vi "VisionTracking.vi"(0 "Refnum in":T1, 5 "Range":cluster{"Lower value":sgl, "Upper value":sgl}={"Lower value"=150.0, "Upper value"=255.0} {"Lower value" scale=0.0..255.0; "Upper value" scale=0.0..255.0}, 7 "Score Limits":T2={"Rect Coverage"=60.0, "X Edge Strength"=40.0, "Y Edge Strength"=60.0, "Center"=75.0, "Outer"=75.0}, 12 "New Image 2":T1, 13 "New Image":T1) -> (4 "Refnum out":T1(plugin-control), 8 "Out Target Info":cluster{"X":dbl, "Y":dbl, "Distance (ft)":dbl}, 10 "Out Cirlcle Info":cluster{"X":dbl, "Y":dbl})   [LabVIEW 2012]
uses:
  <vilib>/vision/Image Controls.llb/IMAQ Image.ctl
  <vilib>/vision/NI_Vision_Development_Module.lvlib
panel:
  out "Circle Info":cluster{dbl, dbl, dbl}[](array[cluster])
  in  "Color Plane":i32(ring)=6 items=["Red", "Green", "Blue", "Hue", "Saturation", "Luminance", "Value", "Intensity"]
  in  "Area Size Limit %":dbl=0.5
  in  "Particle Count Limit":i32=10
  in  "Camera Type":enum16{"206", "1011", "1013"}(ring)
  out "Target Info":T3(array[cluster])
  in  "Annotate":bool=TRUE
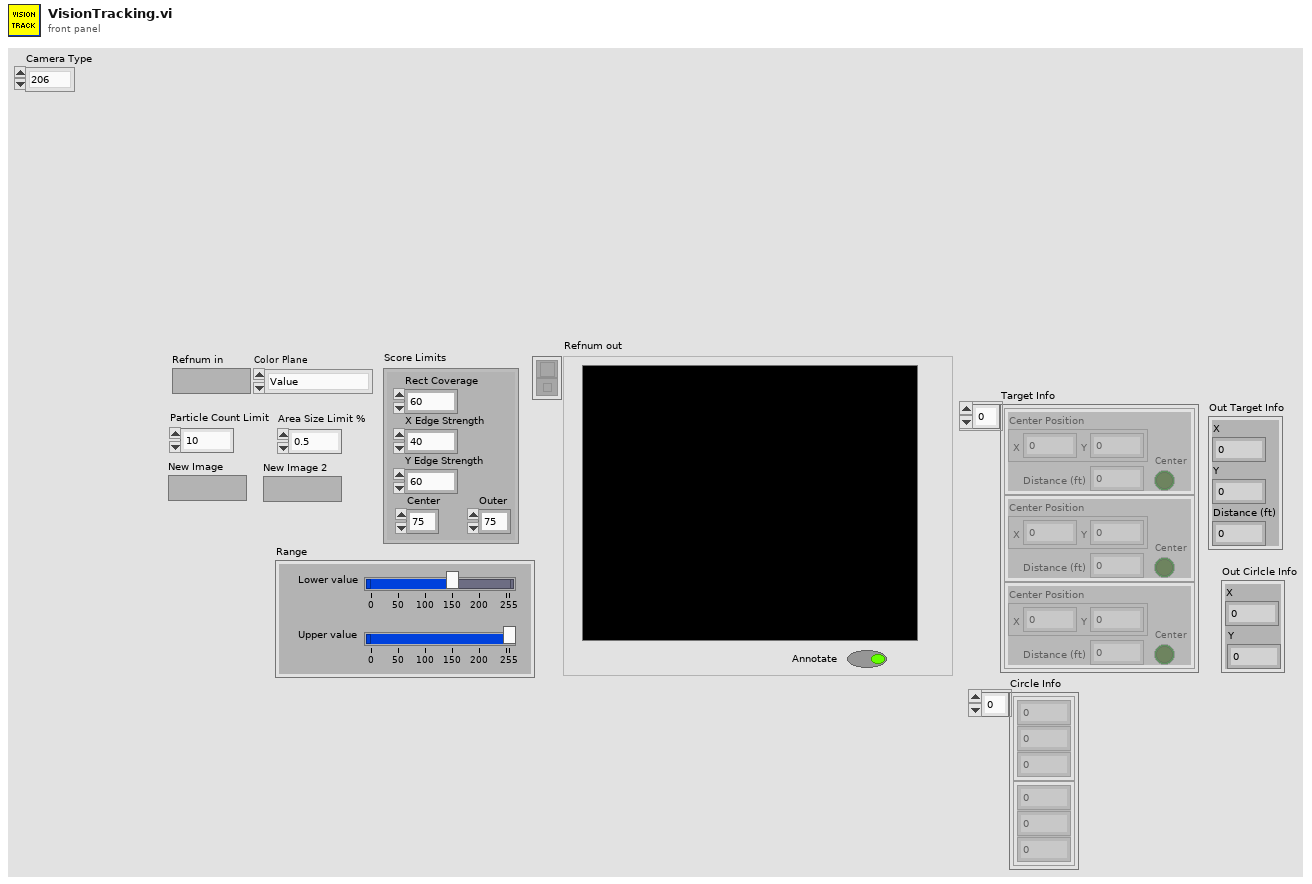
[diagram p1: front panel]
types:
  T1 = typedef "IMAQ Image.ctl" = refnum<image>
  T2 = cluster{"Rect Coverage":dbl, "X Edge Strength":dbl, "Y Edge Strength":dbl, "Center":dbl, "Outer":dbl}
  T3 = cluster{"Center Position":cluster{"X":dbl, "Y":dbl}, "Distance (ft)":dbl, "Center":bool}[]
  T4 = cluster{"Position":cluster{"X":dbl, "Y":dbl}, "Distance (ft)":dbl, bool}[]
  T5 = cluster{cluster{"Left":dbl, "Top":dbl, "Right":dbl, "Bottom":dbl}, "Scores":dbl[], cluster{"Long":dbl, "Short":dbl}}[]
  T6 = cluster{"Target Center (-1 to 1)":cluster{"X":dbl, "Y":dbl}, "Distance (ft)":dbl, "Center Target":bool}
  T7 = cluster{"Target Center (-1 to 1)":cluster{"X":dbl, "Y":dbl}, "Distance (ft)":dbl, "Center Target":bool}[]
  T8 = cluster{"Left":dbl, "Top":dbl, "Right":dbl, "Bottom":dbl}
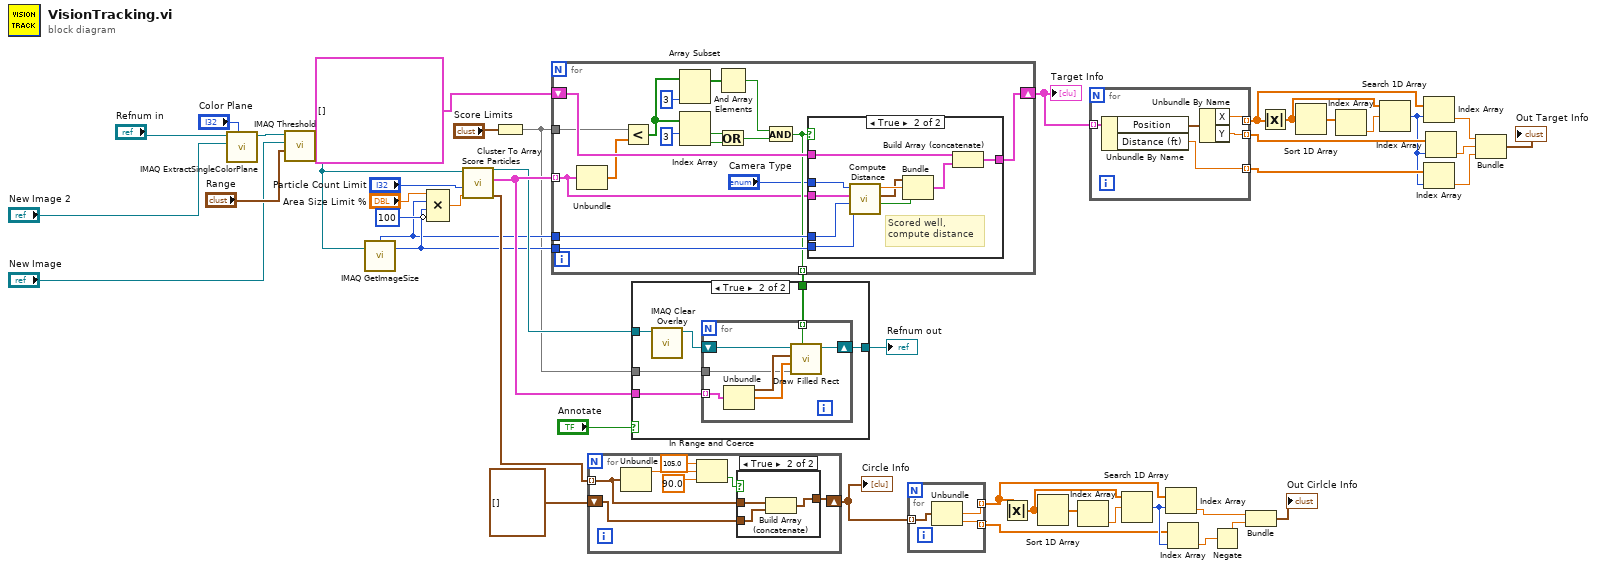
[diagram p0: block diagram]
diagram:
  n1 = call "IMAQ ExtractSingleColorPlane"("Color Plane"="Color Plane", "Image Dst"="New Image 2", "Image Src"="Refnum in") -> ("Image Dst Out"=w14:T1)  [unwired: 1 in, 7 out]
  n2 = call "IMAQ Threshold"("Range"="Range", "Image Dst"="New Image", "Image Src"=w14) -> ("Image Dst Out"=w19:T1)  [unwired: 3 in, 5 out]
  n3 = call "IMAQ GetImageSize"("Image"=w19) -> ("Y Resolution"=w12:i32, "X Resolution"=w11:i32)  [unwired: 3 in, 1 out]
  n4 = Compound Arithmetic op=MULTIPLY("Area Size Limit %", w11, w12, invert 100 ("value")) -> (w17:dbl)
  n5 = call "Score Particles.vi"("Area Size Limit"=w17, "Particle Count Limit"="Particle Count Limit", "Image Refnum in"=w19) -> ("Circle Info"=w23:cluster{dbl, dbl, dbl}[], "Scored Particle Info"=w21:T5, "Image Refnum out"=w20:T1)  [unwired: 6 in]
  n6 = Cluster To Array(cluster="Score Limits") -> (array=w7:dbl[])
  n7 = for {
    shift-right: [w62] -> w45
    shift-left: T4 [] -> [w63]
    tunnel: w11 -> [w61]
    tunnel: w21 -> [w48] mode=indexing
    tunnel: w7 -> [w59]
    tunnel: w12 -> [w58]
    tunnel: [w49] -> w8 mode=indexing
    n8 = Unbundle(w48) -> ("Scores"=w60:dbl[])  [unwired: 2 out]
    n9 = Less?(x=w59, y=w60) -> (x < y?=w55:bool[])
    n10 = Array Subset(array=w55, length=3) -> (w56:bool[])  [unwired: 1 in]
    n11 = Index Array(array=w55, index #1=3 ("length")) -> (element #1=w53:bool, element #2=w52:bool)  [unwired: 1 in]
    n12 = And Array Elements(Boolean array=w56) -> (logical AND=w50:bool)
    n13 = Or(x=w53, y=w52) -> (x .or. y?=w51:bool)
    n14 = And(x=w50, y=w51) -> (x .and. y?=w49:bool)
    n15 = case shown="True" w49 {
      tunnel: w63 -> [w64 w74]
      tunnel: [w64 w73] -> w62
      tunnel: w61 -> [_ w71]
      tunnel: w58 -> [_ w68]
      tunnel: w48 -> [_ w67]
      tunnel: "Camera Type" -> [_ w65]
      frame False {
        # "Didn't score well enough"
      }
      frame True {
        # "Scored well,\ncompute distance"
        n16 = call "Compute Distance.vi"("Y Image Resolution"=w68, "X Image Resolution"=w71, "Particle Scores"=w67, "Camera Type"=w65) -> ("Center Target"=w66:bool, "Target Center (-1 to 1)"=w69:cluster{"X":dbl, "Y":dbl}, "Distance (ft)"=w70:dbl)  [unwired: 5 in]
        n17 = Bundle("Target Center (-1 to 1)"=w69, "Distance (ft)"=w70, "Center Target"=w66) -> (w72:T6)  [unwired: 1 in]
        n18 = Build Array (concatenate)(w74, w72) -> (w73:T7)
      }
    }
  }
  "Target Info" <- w45
  n19 = for {
    tunnel: w23 -> [w77] mode=indexing
    shift-right: [w75] -> w46
    shift-left: cluster{dbl, dbl, dbl}[] [] ("Circle Info") -> [w76]
    n20 = Unbundle(w77) -> (w81:dbl)  [unwired: 2 out]
    n21 = In Range and Coerce(upper limit=105.0, x=w81, lower limit=90.0) -> (In Range?=w78:bool)  [unwired: 1 out]
    n22 = case shown="True" w78 {
      tunnel: w77 -> [_ w85]
      tunnel: w76 -> [w82 w84]
      tunnel: [w82 w83] -> w75
      frame False {
      }
      frame True {
        n23 = Build Array (concatenate)(w85, w84) -> (w83:cluster{dbl, dbl, dbl}[])
      }
    }
  }
  "Circle Info" <- w46
  n24 = case shown="True" "Annotate" {
    tunnel: w20 -> [w86 w92]
    tunnel: [w86 w91] -> w4
    tunnel: w21 -> [_ w89]
    tunnel: w7 -> [_ w88]
    tunnel: w8 -> [_ w87]
    frame False {
    }
    frame True {
      n25 = call "IMAQ Clear Overlay"("Image"=w92) -> ("Image Out"=w90:T1)  [unwired: 2 in, 8 out]
      n26 = for {
        shift-right: [w98] -> w91
        shift-left: w90 -> [w99]
        tunnel: w89 -> [w95] mode=indexing
        tunnel: w88 -> [w94]
        tunnel: w87 -> [w93] mode=indexing
        n27 = Unbundle(w95) -> (w96:T8, "Scores"=w97:dbl[])  [unwired: 1 out]
        n28 = call "Draw Filled Rect.vi"("Limit Passed"=w93, "Limits"=w94, "Scores"=w97, "Bounding Box"=w96, "image in"=w99) -> ("image out"=w98:T1)  [unwired: 6 in]
      }
    }
  }
  "Refnum out" <- w4
  n29 = for {
    tunnel: w46 -> [w102] mode=indexing
    tunnel: [w100] -> w31 mode=indexing
    tunnel: [w101] -> w32 mode=indexing
    n30 = Unbundle(w102) -> (w100:dbl, w101:dbl)  [unwired: 1 out]
  }
  n31 = Absolute Value(x=w31) -> (abs(x)=w29:dbl[])
  n32 = Sort 1D Array(array=w29) -> (sorted array=w28:dbl[])
  n33 = Index Array(array=w28) -> (element=w30:dbl)  [unwired: 1 in]
  n34 = for {
    tunnel: w45 -> [w107] mode=indexing
    tunnel: [w105] -> w41 mode=indexing
    tunnel: [w104] -> w40 mode=indexing
    tunnel: [w103] -> w39 mode=indexing
    n35 = Unbundle By Name(w107) -> ("Position"=w106:cluster{"X":dbl, "Y":dbl}, "Distance (ft)"=w103:dbl)
    n36 = Unbundle By Name(w106) -> ("X"=w105:dbl, "Y"=w104:dbl)
  }
  n37 = Search 1D Array(1D array=w29, element=w30) -> (index of element=w33:i32)  [unwired: 1 in]
  n38 = Index Array(array=w31, index=w33) -> (element=w27:dbl)
  n39 = Index Array(array=w32, index=w33) -> (element=w25:dbl)
  n40 = Negate(x=w25) -> (-x=w24:dbl)
  n41 = Bundle(w27, w24) -> (→"Out Cirlcle Info":cluster{dbl, dbl})  [unwired: 1 in]
  n42 = Absolute Value(x=w41) -> (abs(x)=w43:dbl[])
  n43 = Sort 1D Array(array=w43) -> (sorted array=w44:dbl[])
  n44 = Index Array(array=w44) -> (element=w42:dbl)  [unwired: 1 in]
  n45 = Search 1D Array(1D array=w43, element=w42) -> (index of element=w38:i32)  [unwired: 1 in]
  n46 = Index Array(array=w41, index=w38) -> (element=w37:dbl)
  n47 = Index Array(array=w39, index=w38) -> (element=w35:dbl)
  n48 = Index Array(array=w40, index=w38) -> (element=w36:dbl)
  n49 = Bundle("X"=w37, "Y"=w36, "Distance (ft)"=w35) -> (→"Out Target Info":cluster{"X":dbl, "Y":dbl, "Distance (ft)":dbl})  [unwired: 1 in]
